vi "Display VI.vi"() -> ()   [LabVIEW 2010]
doc: "This VI in conjunction with Generator VI.vi demonstrates how to use network streams to pass data and commands between two running VIs. It displays waveform data that is received from the generator VI and sends commands to update the type of signal that is received.\n\n<B>Note:</B> Requires Generator VI.vi located in the same directory as this VI."
uses:
  resource/objmgr/ni.dex.rc
panel:
  in  "Target IP Address":string="localhost"
  out "Waveform Chart":waveform(dbl)(graph)
  out "error out":errorcluster
  in  "stop":bool
  in  "Signal Type":string(combo)="Sine Waveform"
  # "Instructions:\n1. Open the Generator VI.vi located in the same directory.\n2. Enter target's IP address or DNS name.\n3. Run both VIs at the same time.  Order of starting the VIs is unimportant.\n4. Modify the Signal Type parameter to update the type of waveform generated."
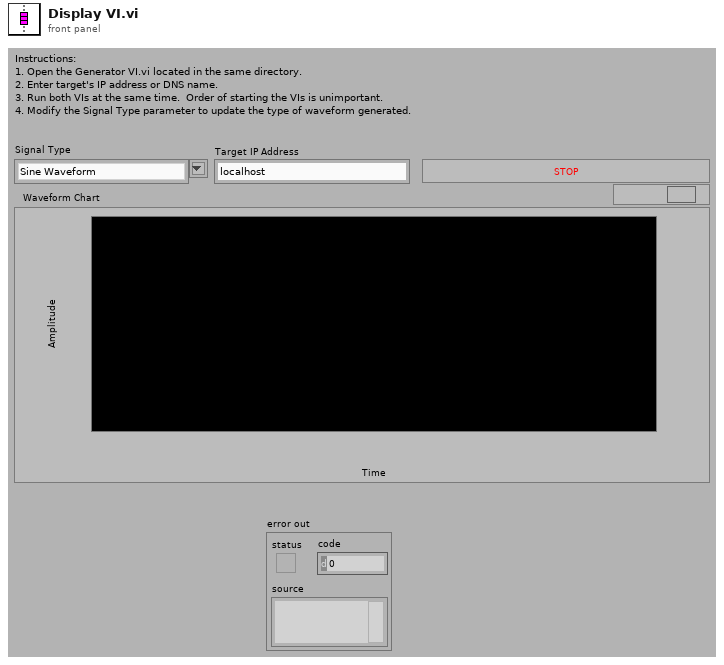
[diagram p1: front panel]
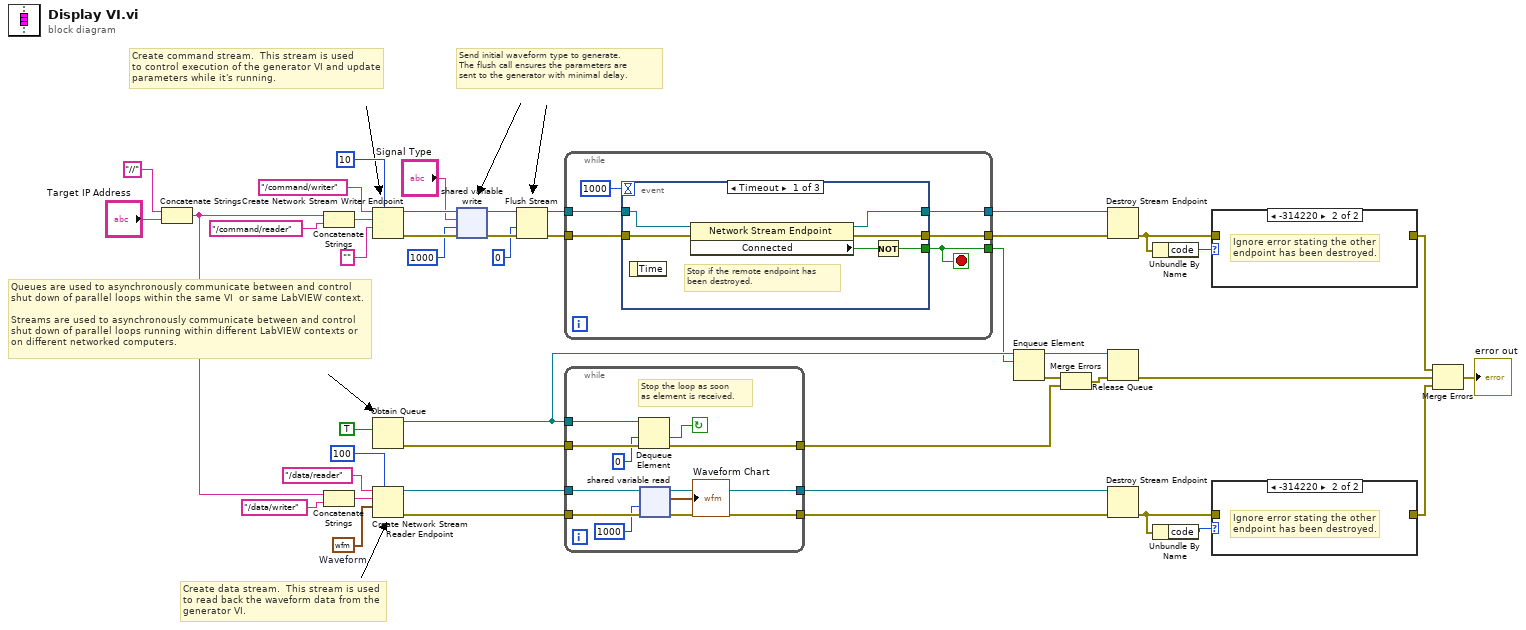
[diagram p0: block diagram]
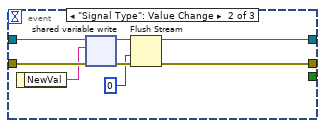
[diagram p4: hidden frame]
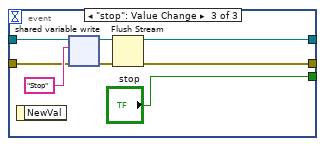
[diagram p5: hidden frame]
diagram:
  w39 = waveform(dbl) {"t0"=timestamp(0 s since 1904-01-01), "dt"=1.0, "Y"=[]}  # Waveform
  # "Send initial waveform type to generate.\nThe flush call ensures the parameters are \nsent to the generator with minimal delay."
  # "Queues are used to asynchronously communicate between and control \nshut down of parallel loops within the same VI  or same LabVIEW context.  \n\nStreams are used to asynchronously communicate between and control \nshut down of parallel loops running within different LabVIEW contexts or \non different networked computers."
  # "Create command stream.  This stream is used\nto control execution of the generator VI and update\nparameters while it's running."
  # "Create data stream.  This stream is used\nto read back the waveform data from the \ngenerator VI."
  n1 = Concatenate Strings("//" ("reader url"), "Target IP Address") -> (w22:string)
  n2 = Concatenate Strings(w22, "/command/reader" ("writer name")) -> (w24:string)
  n3 = Concatenate Strings(w22, "/data/writer" ("reader url")) -> (w25:string)
  n4 = Create Network Stream Writer Endpoint(7:10 ("writer buffer size"), 9:"" ("writer name"), 10:w24, 11:"/command/writer" ("writer name")) -> (0:w31:errorcluster, 3:w33:refnum<k21>)  [unwired: 2 in]
  n5 = Obtain Queue(element data type=TRUE ("stop")) -> (queue out=w16:refnum<queue>, error out=w20:errorcluster)  [unwired: 4 in, 1 out]
  n6 = Create Network Stream Reader Endpoint(7:100 ("reader buffer size"), 9:w39, 10:w25, 11:"/data/reader" ("writer name")) -> (0:w38:errorcluster, 3:w37:refnum<k21>)  [unwired: 2 in]
  n7 = shared-variable-write(w33, w31, "Signal Type", 1000 ("timeout ms")) -> (w32:refnum<k21>, w5:errorcluster)  [unwired: 1 out]
  n8 = Flush Stream(8:w5, 9:0 ("timeout in ms (-1)"), 11:w32) -> (0:w4:errorcluster, 3:w6:refnum<k21>)  [unwired: 1 in, 1 out]
  n9 = while {
    tunnel: w6 -> [w50]
    tunnel: w4 -> [w49]
    tunnel: [w48] -> w42
    tunnel: [w47] -> w41
    tunnel: [w46] -> w13
    stop <- w46 stop-if-true
    n10 = event shown="[0] Timeout" {
      selector: _ -> [_ _ _]
      dyn-events: _ -> [_ _ _]
      timeout: 1000 -> [_ _ _]
      tunnel: w50 -> [w56 w64 w72]
      tunnel: w49 -> [w55 w63 w70]
      tunnel: [w51 w60 w67] -> w48
      tunnel: [w52 w58 w66] -> w47
      tunnel: [w53 _ "stop"] -> w46
      event Timeout {
        # "Stop if the remote endpoint has\nbeen destroyed."
        n11 = event-data() -> ()  [unwired: 1 in, 1 out]
        n12 = property class="Network Stream Endpoint"(reference=w56, error in=w55) -> (reference out=w51:refnum<k21>, error out=w52:errorcluster, "Connected"=w54:bool)
        n13 = Not(x=w54) -> (.not. x?=w53:bool)
      }
      event "Signal Type": Value Change {
        n14 = event-data() -> ("NewVal"=w62:string)  [unwired: 1 in]
        n15 = shared-variable-write(w64, w63, w62) -> (w61:refnum<k21>, w59:errorcluster)  [unwired: 1 in, 1 out]
        n16 = Flush Stream(8:w59, 9:0 ("timeout in ms (-1)"), 11:w61) -> (0:w58:errorcluster, 3:w60:refnum<k21>)  [unwired: 1 in, 1 out]
      }
      event "stop": Value Change {
        n17 = event-data() -> ()  [unwired: 1 in, 1 out]
        n18 = shared-variable-write(w72, w70, "Stop" ("writer name")) -> (w69:refnum<k21>, w68:errorcluster)  [unwired: 1 in, 1 out]
        n19 = Flush Stream(8:w68, 11:w69) -> (0:w66:errorcluster, 3:w67:refnum<k21>)  [unwired: 2 in, 1 out]
      }
    }
  }
  n20 = while {
    tunnel: w38 -> [w83]
    tunnel: w37 -> [w82]
    tunnel: [w80] -> w36
    tunnel: [w79] -> w35
    tunnel: w16 -> [w76]
    tunnel: w20 -> [w77]
    tunnel: [w73] -> w15
    stop <- w74 continue-if-true
    # "Stop the loop as soon \nas element is received."
    n21 = Dequeue Element(queue=w76, timeout in ms (-1)=0, error in (no error)=w77) -> (timed out?=w74:bool, error out=w73:errorcluster)  [unwired: 2 out]
    n22 = shared-variable-read(w82, w83, 1000 ("timeout ms")) -> (w79:refnum<k21>, w80:errorcluster, →"Waveform Chart":waveform(dbl))  [unwired: 1 out]
  }
  n23 = Enqueue Element(queue=w16, element=w13) -> (queue out=w19:refnum<queue>, error out=w18:errorcluster)  [unwired: 2 in, 1 out]
  n24 = Merge Errors(w18, w15) -> (w17:errorcluster)
  n25 = Destroy Stream Endpoint(8:w41, 11:w42) -> (0:w11:errorcluster)
  n26 = Release Queue(queue=w19, error in (no error)=w17) -> (error out=w14:errorcluster)  [unwired: 1 in, 2 out]
  n27 = Destroy Stream Endpoint(8:w36, 11:w35) -> (0:w8:errorcluster)
  n28 = Unbundle By Name(w11) -> ("code"=w12:i32)
  n29 = Unbundle By Name(w8) -> ("code"=w9:i32)
  n30 = case shown="-314220" w12 {
    tunnel: w11 -> [w84 _]
    tunnel: [w84 _] -> w10
    frame 0, Default {
    }
    frame -314220 {
      # "Ignore error stating the other\nendpoint has been destroyed."
    }
  }
  n31 = case shown="-314220" w9 {
    tunnel: w8 -> [w85 _]
    tunnel: [w85 _] -> w7
    frame 0, Default {
    }
    frame -314220 {
      # "Ignore error stating the other\nendpoint has been destroyed."
    }
  }
  n32 = Merge Errors(w10, w14, w7) -> (→"error out":errorcluster)
